vi "Check for Thread Errors.vi"(8 "error in (no error)":errorcluster, 11 "Framework in":refnum<class "Framework.lvclass">) -> (0 "error out":errorcluster, 3 "Framework out":refnum<class "Framework.lvclass">)   [LabVIEW 2017, in "DSF Core.lvlib" / "Framework.lvclass"]
uses:
  Framework.lvclass
  Framework.lvclass/Framework.ctl
  Thread Manager/Thread Manager.lvclass
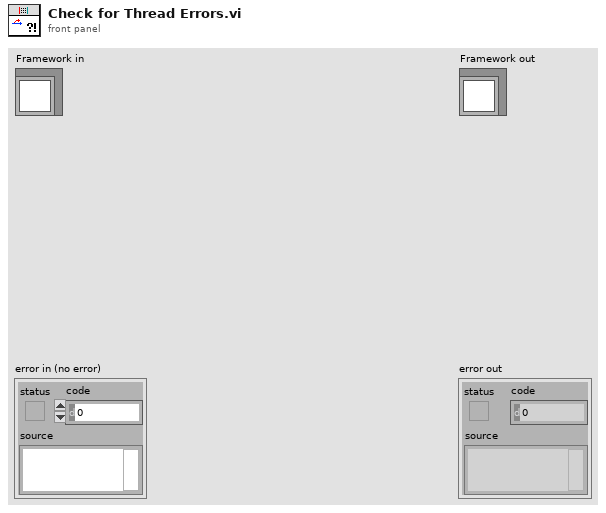
[diagram p1: front panel]
types:
  T1 = typedef "DSF Core.lvlib/Thread.lvclass/Thread State.ctl" = enum8{"Idle", "Running", "Error", "Shut Down"}
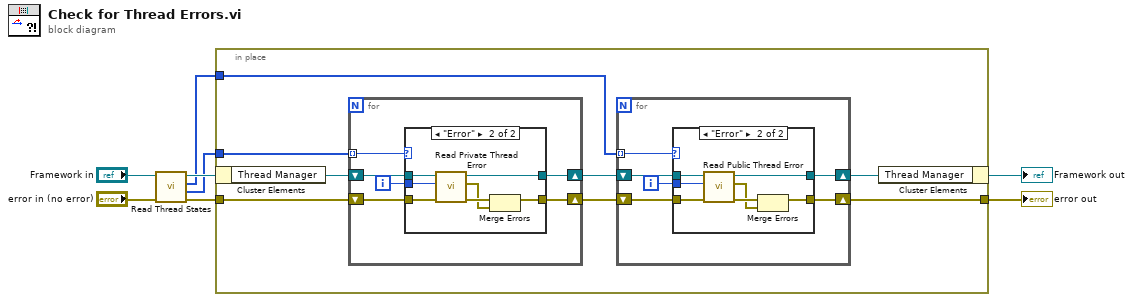
[diagram p0: block diagram]
diagram:
  n1 = call "Read Thread States.vi"("error in (no error)"="error in (no error)", "Framework in"="Framework in") -> ("error out"=w4:errorcluster, "public thread states"=w1:T1[], "private thread states"=w2:T1[], "Framework out"=w3:refnum<class "Framework.lvclass">)  [unwired: 6 in]
  n2 = in-place {
    in-place-border: w4 -> [w15]
    in-place-border: [w10] -> w7
    in-place-border: w2 -> [w9]
    in-place-border: w1 -> [w14]
    n3 = in-place-cluster #1(w3) -> ("Thread Manager"=w16:refnum<class "Thread Manager.lvclass">)
    n4 = for {
      shift-right: [w34] -> w12
      shift-left: w16 -> [w37]
      shift-right: [w35] -> w13
      shift-left: w15 -> [w36]
      tunnel: w14 -> [w33] mode=indexing
      i -> [w32]
      n5 = case shown="\"Error\"" w33 {
        tunnel: w37 -> [w39 w46]
        tunnel: w36 -> [w38 w45]
        tunnel: [w38 w42] -> w35
        tunnel: [w39 w41] -> w34
        tunnel: w32 -> [_ w40]
        frame Default {
        }
        frame "Error" {
          n6 = call "Read Private Thread Error.vi"("error in (no error)"=w45, "thread index"=w40, "Thread Manager in"=w46) -> ("error out"=w44:errorcluster, "thread error"=w43:errorcluster, "Thread Manager out"=w41:refnum<class "Thread Manager.lvclass">)  [unwired: 6 in]
          n7 = Merge Errors(w44, w43) -> (w42:errorcluster)
        }
      }
    }
    n8 = for {
      shift-right: [w19] -> w11
      shift-left: w12 -> [w22]
      shift-right: [w20] -> w10
      shift-left: w13 -> [w21]
      tunnel: w9 -> [w18] mode=indexing
      i -> [w17]
      n9 = case shown="\"Error\"" w18 {
        tunnel: w22 -> [w24 w30]
        tunnel: w21 -> [w23 w29]
        tunnel: [w23 w31] -> w20
        tunnel: [w24 w28] -> w19
        tunnel: w17 -> [_ w26]
        frame Default {
        }
        frame "Error" {
          n10 = call "Read Public Thread Error.vi"("error in (no error)"=w29, "thread index"=w26, "Thread Manager in"=w30) -> ("error out"=w27:errorcluster, "thread error"=w25:errorcluster, "Thread Manager out"=w28:refnum<class "Thread Manager.lvclass">)  [unwired: 6 in]
          n11 = Merge Errors(w27, w25) -> (w31:errorcluster)
        }
      }
    }
    n12 = in-place-cluster #1("Thread Manager"=w11) -> (→"Framework out":refnum<class "Framework.lvclass">)
  }
  "error out" <- w7
